vi "VMI_data_sort.vi"(4 "Power Err":dbl[][](array[numeric]), 5 "Numeric":i32, 6 "xaxis":i32[][](array[numeric]), 7 "Histogram":i32[][](array[numeric]), 9 "Powers":dbl[][](array[numeric]), 10 "Peak Array":cluster{"X":sgl, "Y":sgl}[][](array[cluster]), 11 "Data":T1[](array[typedef])) -> (2 "Data Out":T1[](array[typedef]), 3 "HistArray":dbl[][][](array[numeric]))   [LabVIEW 2018]
uses:
  Type defs/VMI_peak_out.ctl
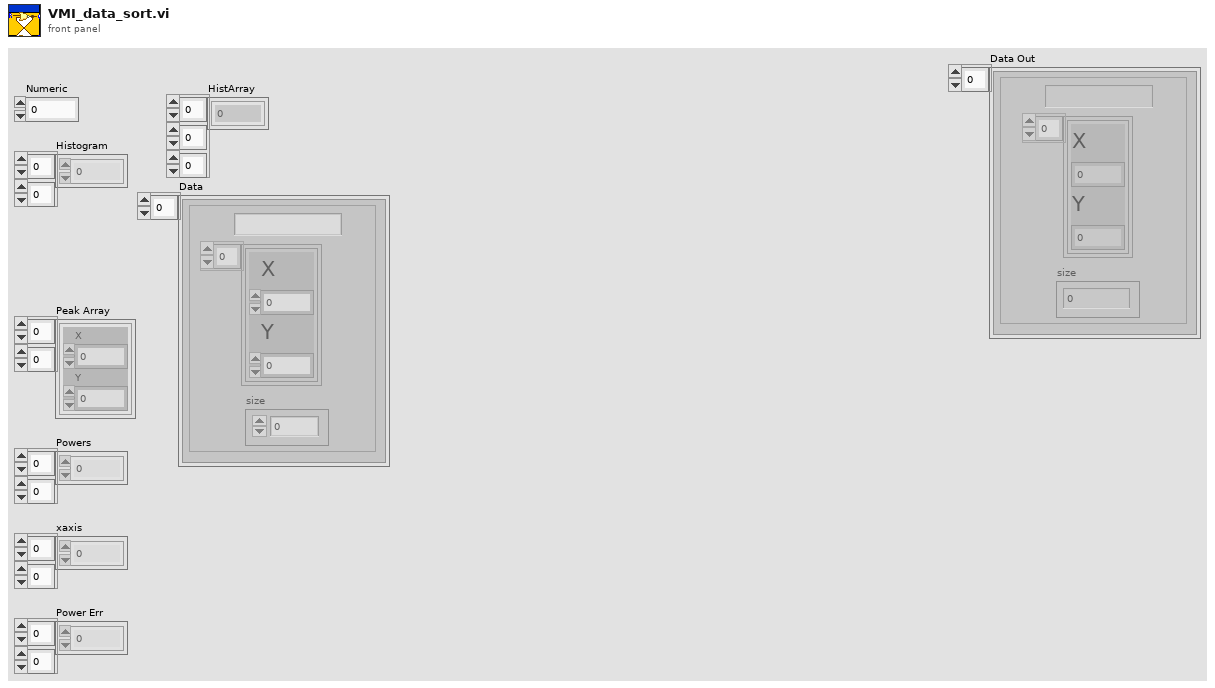
[diagram p1: front panel]
types:
  T1 = typedef "VMI_peak_out.ctl" = cluster{"Peaks":cluster{"X":sgl, "Y":sgl}[], "size":i32, "Title":string}
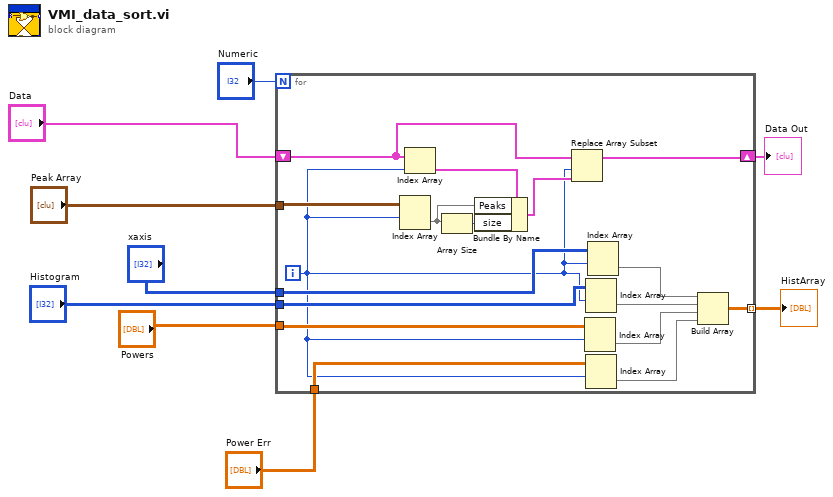
[diagram p0: block diagram]
diagram:
  n1 = for {
    N: "Numeric" -> [_]
    tunnel: "Peak Array" -> [w23]
    tunnel: "Histogram" -> [w20]
    tunnel: "Powers" -> [w18]
    tunnel: "Power Err" -> [w16]
    tunnel: [w24] -> w7 mode=indexing
    tunnel: "xaxis" -> [w22]
    shift-right: [w11] -> w1
    shift-left: "Data" -> [w10]
    i -> [w14]
    n2 = Index Array(array=w23, index (row)=w14) -> (element=w13:cluster{"X":sgl, "Y":sgl}[])  [unwired: 1 in]
    n3 = Index Array(array=w10, index=w14) -> (element=w26:T1)
    n4 = Array Size(array=w13) -> (size(s)=w12:i32)
    n5 = Bundle By Name(cluster=w26, "Peaks"=w13, "size"=w12) -> (w25:T1)
    n6 = Replace Array Subset(array=w10, new element=w25, index=w14) -> (w11:T1[])
    n7 = Index Array(array=w18, index (row)=w14) -> (element=w17:dbl[])  [unwired: 1 in]
    n8 = Index Array(array=w20, index (row)=w14) -> (element=w19:i32[])  [unwired: 1 in]
    n9 = Index Array(array=w16, index (row)=w14) -> (element=w15:dbl[])  [unwired: 1 in]
    n10 = Index Array(array=w22, index (row)=w14) -> (element=w21:i32[])  [unwired: 1 in]
    n11 = Build Array(w21, w19, w17, w15) -> (w24:dbl[][])
  }
  "HistArray" <- w7
  "Data Out" <- w1
